vi "getSamplingMode.vi"(8 "error in (no error)":errorcluster, 11 "Instrument.LockinAPI in":refnum<class "Instrument.LockinAPI.lvclass">) -> (0 "error out":errorcluster, 2 "Fs Mode":T1, 3 "Instrument.LockinAPI out":refnum<class "Instrument.LockinAPI.lvclass">)   [LabVIEW 2019, in "Instrument.LockinAPI.lvclass"]
doc: "API to get the configured sampling mode\n\nIf address=\"\", this API reads from localhost\nIf address is remote lockin, you need to add this computer to allowed whitelist on the lockin computer you are trying to access."
uses:
  Instrument.LockinAPI.lvclass
  Typedefs/LockinAPI.Sampling.FsMode--enum.ctl
  Typedefs/LockinAPI.commands--Enum.ctl
  Instrument/Instrument.lvclass
  C:/Users/patrick/Documents/GitHub/Instrument-Framework/lvsrc/Framework/Instrument/Instrument.lvclass
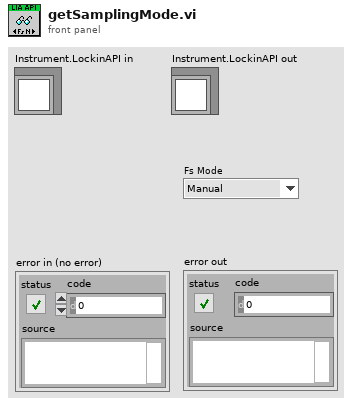
[diagram p1: front panel]
types:
  T1 = typedef "Instrument.LockinAPI.lvclass/LockinAPI.Sampling.FsMode--enum.ctl" = enum16{"Manual", "Auto Fs", "Max Fs"}
  T2 = typedef "Instrument.LockinAPI.lvclass/LockinAPI.commands--Enum.ctl" = enum16{"setAI", "setAO", "setAO_Amplitude", "setAO_DC", "setAO_Frequency", "setAO_Phase", "setAO_Function", "setAO_I+", "setREF", "setREF_Frequency", "setREF_Phase", "setREF_TC", "setREF_Roll-Off", "setDAQ", "setSampling", "setOffset", "setState", "getState", "getAO", "getAI", "getResults", "getSampling", "getAOconfig", "getREFconfig", "setInputGain", "setOutputGain", "getInputGain", "getOutputGain", "setSamplingMode", "getSamplingMode", "setSweep", "setSweepTime", "setSweepTable", "getStatus", "getSweepResults", "getSweepWaveforms", "startSweep", "stopSweep", "setAUX", "getAUX"}
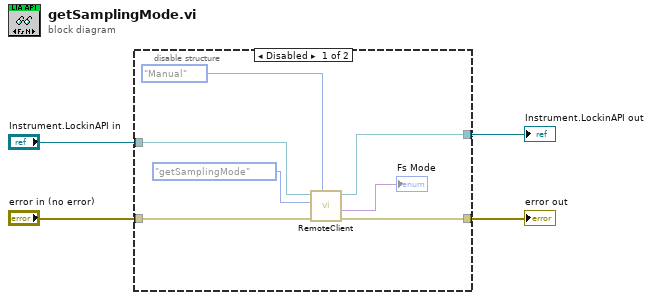
[diagram p0: block diagram]
diagram:
  n1 = disable-structure shown="Disabled" {
    disable-tunnel: [w10 w13] -> w4
    disable-tunnel: "Instrument.LockinAPI in" -> [w8 w12]
    disable-tunnel: [w7 w12] -> w2
    disable-tunnel: "error in (no error)" -> [w11 w13]
    frame Disabled {
      n2 = call "RemoteClient.vi"("timeout (ms) [500]"=LockinAPI.Sampling.FsMode--enum."Manual" ("Fs Mode"), "error in (no error)"=w11, "Command in"=LockinAPI.commands--Enum."getSamplingMode" ("Command"), "Instrument in"=w8) -> ("error out"=w10:errorcluster, "Data out"=→"Fs Mode":variant, "Instrument out"=w7:refnum<class "Instrument.LockinAPI.lvclass">)  [unwired: 4 in, 1 out]
    }
    frame Enabled {
    }
  }
  "error out" <- w4
  "Instrument.LockinAPI out" <- w2
